vi "Set range.vi"(0 "RBD9103":T2, 2 "Range":T1 items=["Auto range", "2 nA", "20 nA", "200 nA", "2 uA", "20 uA", "200 uA", "2 mA"], 5 "error in":errorcluster) -> (14 "RBD9103 out":T2, 16 "Range out":T1 items=["Auto range", "2 nA", "20 nA", "200 nA", "2 uA", "20 uA", "200 uA", "2 mA"], 19 "error out":errorcluster)   [LabVIEW 2017]
uses:
  Operation type.ctl
  Range.ctl
  GenericDataEvent/GenericEvent.ctl
  RBD9103.ctl
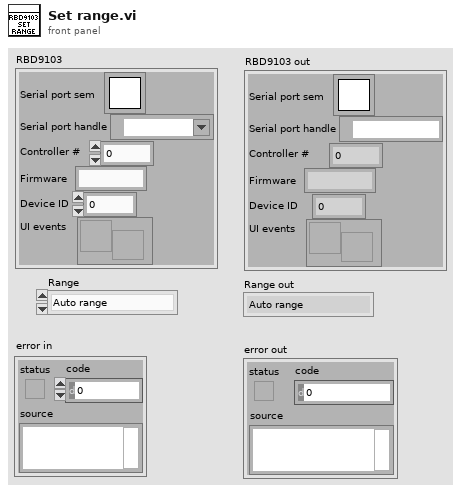
[diagram p1: front panel]
types:
  T1 = typedef "Range.ctl" = u16
  T2 = typedef "RBD9103.ctl" = cluster{"Serial port sem":T3, "Serial port handle":refnum<visa-resource-name>, "Controller #":u8, "Firmware":string, "Device ID":i32, "UI events":T4}
  T3 = typedef "Semaphore RefNum" = refnum<k1>
  T4 = typedef "GenericEvent.ctl" = refnum<user-event>
  T5 = typedef "Operation type.ctl" = enum16{"Write&Read", "Read only", "Write only", "Read only multiply"}
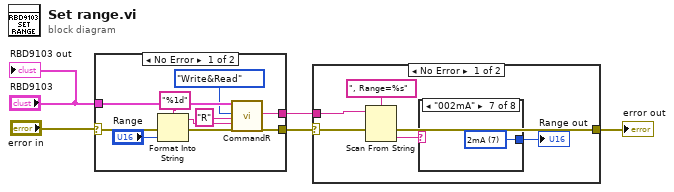
[diagram p0: block diagram]
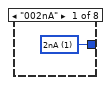
[diagram p2: hidden frame]
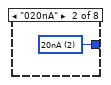
[diagram p3: hidden frame]
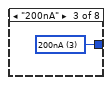
[diagram p4: hidden frame]
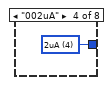
[diagram p5: hidden frame]
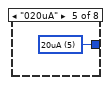
[diagram p6: hidden frame]
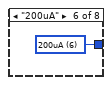
[diagram p7: hidden frame]
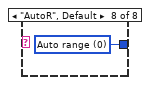
[diagram p8: hidden frame]
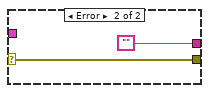
[diagram p10: hidden frame]
diagram:
  n1 = case shown="No Error" "error in" {
    selector: "error in" -> [w9 w17]
    tunnel: [w14 w17] -> w3
    tunnel: "RBD9103" -> [w15 _]
    tunnel: [w12 ""] -> w1
    frame No Error {
      n2 = Format Into String(format string="%1d", error in=w9, "Range") -> (resulting string=w6:string, error out=w8:errorcluster)  [unwired: 1 in]
      n3 = call "CommandR.vi"("RBD9103"=w15, "Operation"=Operation_type."Write&Read" ("Operation type"), "Command"="R", "Data"=w6, "error in"=w8) -> ("Answer"=w12:string, "error out"=w14:errorcluster)  [unwired: 11 in, 2 out]
    }
    frame Error {
    }
  }
  n4 = case shown="No Error" w3 {
    selector: w3 -> [w22 w32]
    tunnel: [w20 w32] -> w2
    tunnel: w1 -> [w21 _]
    frame No Error {
      n5 = Scan From String(format string=", Range=%s", input string=w21, error in=w22) -> (error out=w20:errorcluster, output 1=w19:string)  [unwired: 2 in, 2 out]
      n6 = case shown="\"002mA\"" w19 {
        tunnel: [w24 w25 w26 w27 w28 w29 w30 w31] -> w18
        frame "002nA" {
          w24 = T1 1 items=["Auto range", "2nA", "20nA", "200nA", "2uA", "20uA", "200uA", "2mA"] ("Range out")
        }
        frame "020nA" {
          w25 = T1 2 items=["Auto range", "2nA", "20nA", "200nA", "2uA", "20uA", "200uA", "2mA"] ("Range out")
        }
        frame "200nA" {
          w26 = T1 3 items=["Auto range", "2nA", "20nA", "200nA", "2uA", "20uA", "200uA", "2mA"] ("Range out")
        }
        frame "002uA" {
          w27 = T1 4 items=["Auto range", "2nA", "20nA", "200nA", "2uA", "20uA", "200uA", "2mA"] ("Range out")
        }
        frame "020uA" {
          w28 = T1 5 items=["Auto range", "2nA", "20nA", "200nA", "2uA", "20uA", "200uA", "2mA"] ("Range out")
        }
        frame "200uA" {
          w29 = T1 6 items=["Auto range", "2nA", "20nA", "200nA", "2uA", "20uA", "200uA", "2mA"] ("Range out")
        }
        frame "002mA" {
          w30 = T1 7 items=["Auto range", "2nA", "20nA", "200nA", "2uA", "20uA", "200uA", "2mA"] ("Range out")
        }
        frame "AutoR", Default {
          w31 = T1 0 items=["Auto range", "2nA", "20nA", "200nA", "2uA", "20uA", "200uA", "2mA"] ("Range out")
        }
      }
      "Range out" <- w18
    }
    frame Error {
    }
  }
  "error out" <- w2
  "RBD9103 out" <- "RBD9103"
